vi "Read Y Trace.vi"(7 "array length":i32=1 caption="array length (1)" format="%.0g", 8 "error in (no error)":errorcluster {"code" format="%.0x"}, 9 "maximum time":i32=1000 caption="maximum time (1000 ms)" format="%#.0f", 10 "trace name":string="Trace1" caption="trace name (Trace1)", 11 "instrument handle":refnum<k15>) -> (0 "error out":errorcluster {"code" format="%.0x"}, 1 "actual points":i32 format="%.0g", 2 "amplitude":dbl[](array[numeric]), 3 "instrument handle out":refnum<k15>)   [LabVIEW 2009, in "Keysight XSAn.lvlib"]
doc: "This VI initiates a signal acquisition, waits for the completion, and returns the trace as amplitude array.\n\nSupported Models: M9290A, N8973B, N8974B, N8975B, N8976B, N9000A, N9000B, N9010A, N9010B, N9020A, N9020B, N9030A, N9030B, N9038A, N9040B, N9041B, SPN9003A, SPN9026A"
uses:
  <instrlib>/Keysight XSAn/Keysight XSAn.lvlib
  AgXSAn.dll
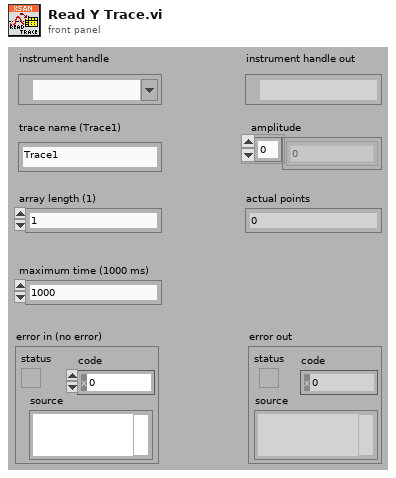
[diagram p1: front panel]
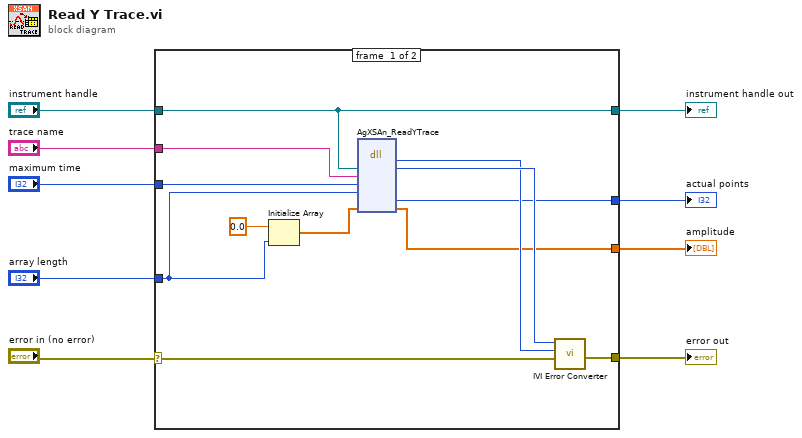
[diagram p0: block diagram]
diagram:
  n1 = case shown="No Error" "error in (no error)" {
    selector: "error in (no error)" -> [w17 w23]
    tunnel: [w18 w23] -> w8
    tunnel: "instrument handle" -> [w12 w22]
    tunnel: "array length" -> [w15 _]
    tunnel: "maximum time" -> [w14 _]
    tunnel: "trace name" -> [w13 _]
    tunnel: [w12 w22] -> w3
    tunnel: [w11 _] -> w2
    tunnel: [w10 _] -> w1
    frame #0 {
      n2 = Initialize Array(0.0, w15) -> (w20:dbl[])
      n3 = dll-call lib="AgXSAn**.dll" fn="AgXSAn_ReadYTrace" ("LabVIEW:IviSpecAn_ReadYTrace")("instrument handle"=w12, "trace name"=w13, "maximum time (ms)"=w14, "array length"=w15, "amplitude"=w20) -> ("Status"=w16:i32, "instrument handle"=w19:u32, "actual points"=w11:i32, "amplitude"=w10:dbl[])  [unwired: 6 in, 3 out]
      n4 = call <instrlib>:"IVI Error Converter.vi"("error in (no error)"=w17, "IVI error code (0)"=w16, "instrument handle"=w19) -> ("error out"=w18:errorcluster)  [unwired: 7 in, 1 out]
    }
    frame #1 {
    }
  }
  "error out" <- w8
  "instrument handle out" <- w3
  "actual points" <- w2
  "amplitude" <- w1
